vi "Message-Enqueuer References Control Label.vi"() -> (0 "Message-Enqueuer References Control Label":string)   [LabVIEW 2018, in "Scripting.lvlib"]
uses:
  Scripting.lvlib
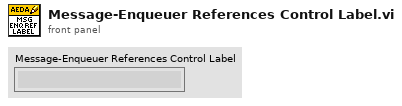
[diagram p1: front panel]
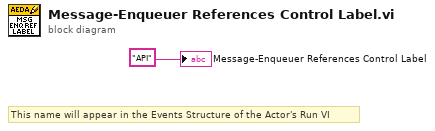
[diagram p0: block diagram]
diagram:
  # "This name will appear in the Events Structure of the Actor's Run VI"
  "Message-Enqueuer References Control Label" <- "API" ("y")
